vi "Global 1.vi"() -> ()   [LabVIEW 2011]
panel:
  in  "Autonomous mode":T1(ring)
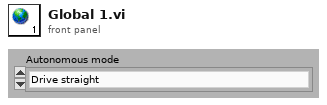
[diagram p1: front panel]
types:
  T1 = enum16{"Drive straight", "Drive straight and follow line", "Drive and follow fork left", "Drive and follow fork right"}
diagram:
